vi "postPubDataUE.vi"(6 "newValue (T)":bool=TRUE, 8 "error in (no error)":errorcluster, 9 "value":variant, 10 "pubDataSV":T1=enum."LoopTime_ms", 11 "PubSubDataEvent in":refnum<class "PubSubDataEvent.lvclass">) -> (0 "error out":errorcluster, 3 "PubSubDataEvent out":refnum<class "PubSubDataEvent.lvclass">)   [LabVIEW 2016, in "PubSubDataEvent.lvclass"]
uses:
  PubSubDataEvent.lvclass
  Typedefs/PubDataSV.ctl
  PubSubDataEvent.lvclass/PubSubDataEvent.ctl
  Typedefs/StateValue.ctl
  Typedefs/RejectedCommand.ctl
  Typedefs/CommandValue.ctl
  ComponentTemplateCore/ComponentModel/ComponentModel/Typedefs/ComponentStateValues.ctl
  Typedefs/EXATypedefs.lvlib
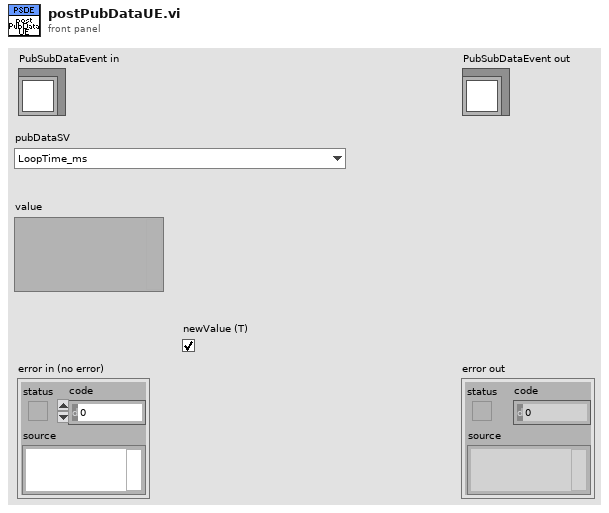
[diagram p1: front panel]
types:
  T1 = typedef "EXATypedefs.lvlib/PubDataSV.ctl" = enum16{"DetailedState", "ErrorCode", "Heartbeat", "LoopTime_ms", "LoopTimeOutOfRange", "RejectedCommand", "SummaryState", "Timestamp"}
  T2 = typedef "EXATypedefs.lvlib/PubDataEvents.ctl" = cluster{"DetailedState":refnum<user-event>, "ErrorCode":refnum<user-event>, "Heartbeat":refnum<user-event>, "LoopTime_ms":refnum<user-event>, "LoopTimeOutOfRange":refnum<user-event>, "RejectedCommand":refnum<user-event>, "SummaryState":refnum<user-event>, "Timestamp":refnum<user-event>}
  T3 = typedef "EXATypedefs.lvlib/StateValue.ctl" = enum16{"DisabledState", "EnabledState", "FaultState", "OffState", "StandbyState"}
  T4 = typedef "EXATypedefs.lvlib/RejectedCommand.ctl" = cluster{"CommandValue":T5, "StateValue":T3, "Time Stamp":timestamp}
  T5 = typedef "EXATypedefs.lvlib/CommandValue.ctl" = enum16{"ClearError", "Disable", "Enable", "Exit", "GoToStandby", "OnHeartbeat", "OnIncomingMessagingError", "OnInterrupt", "Start"}
  T6 = typedef "ComponentStateValues.ctl" = enum16{"Off", "Standby", "Enabled", "Disabled", "Fault"}
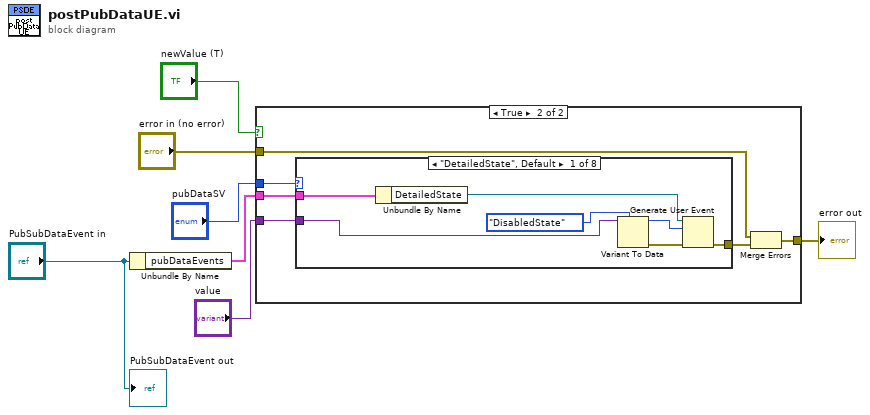
[diagram p0: block diagram]
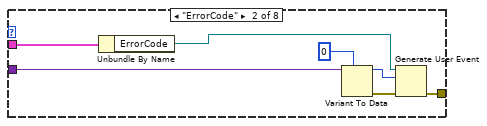
[diagram p3: hidden frame]
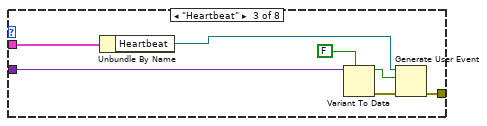
[diagram p4: hidden frame]
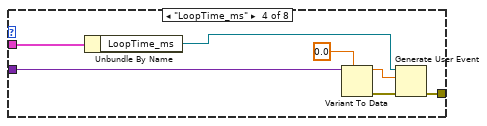
[diagram p5: hidden frame]
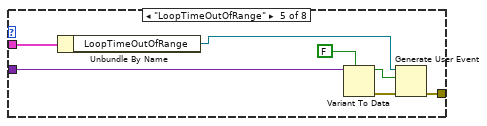
[diagram p6: hidden frame]
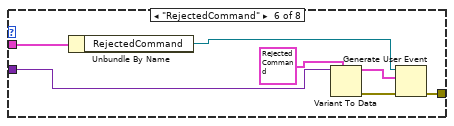
[diagram p7: hidden frame]
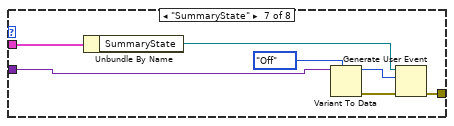
[diagram p8: hidden frame]
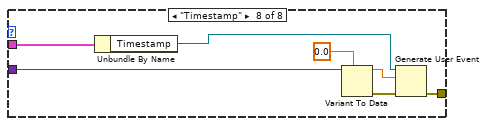
[diagram p9: hidden frame]
diagram:
  n1 = Unbundle By Name("PubSubDataEvent in") -> ("pubDataEvents"=w6:T2)
  n2 = case shown="True" "newValue (T)" {
    tunnel: "pubDataSV" -> [_ w11]
    tunnel: "value" -> [_ w10]
    tunnel: "error in (no error)" -> [w8 w13]
    tunnel: [w8 w14] -> w4
    tunnel: w6 -> [_ w12]
    frame False {
    }
    frame True {
      n3 = case shown="\"DetailedState\", Default" w11 {
        tunnel: w12 -> [w21 w28 w35 w42 w49 w56 w63 w70]
        tunnel: w10 -> [w19 w26 w33 w40 w47 w54 w61 w68]
        tunnel: [w18 w25 w32 w39 w46 w53 w60 w67] -> w9
        frame "DetailedState", Default {
          n4 = Unbundle By Name(w21) -> ("DetailedState"=w20:refnum<user-event>)
          n5 = Variant To Data(type=StateValue."DisabledState" ("event data"), Variant=w19) -> (data=w16:T3, error out=w15:errorcluster)  [unwired: 1 in]
          n6 = Generate User Event(user event=w20, event data cluster=w16, error in=w15) -> (error out=w18:errorcluster)  [unwired: 1 in, 1 out]
        }
        frame "ErrorCode" {
          n7 = Unbundle By Name(w28) -> ("ErrorCode"=w27:refnum<user-event>)
          n8 = Variant To Data(type=0 ("event data"), Variant=w26) -> (data=w22:i32, error out=w24:errorcluster)  [unwired: 1 in]
          n9 = Generate User Event(user event=w27, event data cluster=w22, error in=w24) -> (error out=w25:errorcluster)  [unwired: 1 in, 1 out]
        }
        frame "Heartbeat" {
          n10 = Unbundle By Name(w35) -> ("Heartbeat"=w34:refnum<user-event>)
          n11 = Variant To Data(type=FALSE ("event data"), Variant=w33) -> (data=w29:bool, error out=w31:errorcluster)  [unwired: 1 in]
          n12 = Generate User Event(user event=w34, event data cluster=w29, error in=w31) -> (error out=w32:errorcluster)  [unwired: 1 in, 1 out]
        }
        frame "LoopTime_ms" {
          n13 = Unbundle By Name(w42) -> ("LoopTime_ms"=w41:refnum<user-event>)
          n14 = Variant To Data(type=0.0 ("event data"), Variant=w40) -> (data=w36:dbl, error out=w38:errorcluster)  [unwired: 1 in]
          n15 = Generate User Event(user event=w41, event data cluster=w36, error in=w38) -> (error out=w39:errorcluster)  [unwired: 1 in, 1 out]
        }
        frame "LoopTimeOutOfRange" {
          n16 = Unbundle By Name(w49) -> ("LoopTimeOutOfRange"=w48:refnum<user-event>)
          n17 = Variant To Data(type=FALSE ("event data"), Variant=w47) -> (data=w43:bool, error out=w45:errorcluster)  [unwired: 1 in]
          n18 = Generate User Event(user event=w48, event data cluster=w43, error in=w45) -> (error out=w46:errorcluster)  [unwired: 1 in, 1 out]
        }
        frame "RejectedCommand" {
          n19 = Unbundle By Name(w56) -> ("RejectedCommand"=w55:refnum<user-event>)
          n20 = Variant To Data(type=T4 {"CommandValue"=enum."ClearError", "StateValue"=enum."DisabledState", "Time Stamp"=timestamp(0 s since 1904-01-01)} ("event data"), Variant=w54) -> (data=w50:T4, error out=w52:errorcluster)  [unwired: 1 in]
          n21 = Generate User Event(user event=w55, event data cluster=w50, error in=w52) -> (error out=w53:errorcluster)  [unwired: 1 in, 1 out]
        }
        frame "SummaryState" {
          n22 = Unbundle By Name(w63) -> ("SummaryState"=w62:refnum<user-event>)
          n23 = Variant To Data(type=ComponentStateValues."Off" ("event data"), Variant=w61) -> (data=w57:T6, error out=w59:errorcluster)  [unwired: 1 in]
          n24 = Generate User Event(user event=w62, event data cluster=w57, error in=w59) -> (error out=w60:errorcluster)  [unwired: 1 in, 1 out]
        }
        frame "Timestamp" {
          n25 = Unbundle By Name(w70) -> ("Timestamp"=w69:refnum<user-event>)
          n26 = Variant To Data(type=0.0 ("event data"), Variant=w68) -> (data=w64:dbl, error out=w66:errorcluster)  [unwired: 1 in]
          n27 = Generate User Event(user event=w69, event data cluster=w64, error in=w66) -> (error out=w67:errorcluster)  [unwired: 1 in, 1 out]
        }
      }
      n28 = Merge Errors(w13, w9) -> (w14:errorcluster)
    }
  }
  "error out" <- w4
  "PubSubDataEvent out" <- "PubSubDataEvent in"
